vi "Example2.vi"() -> ()   [LabVIEW 2021]
doc: "Example of data acces and data flow in OOP in LabVIEW. Comments in Polish."
uses:
  Spaceship/Spaceship.lvclass
panel:
  out "Error Out 3":errorcluster
  out "Message Out 2":string
  out "Message Out":string
  in  "Spaceship.lvclass 2":refnum<class "Spaceship.lvclass">
  out "Error Out":errorcluster
  out "Error Out 2":errorcluster
  out "ID 2":string
  out "ID":string
  in  "Spaceship.lvclass":refnum<class "Spaceship.lvclass">
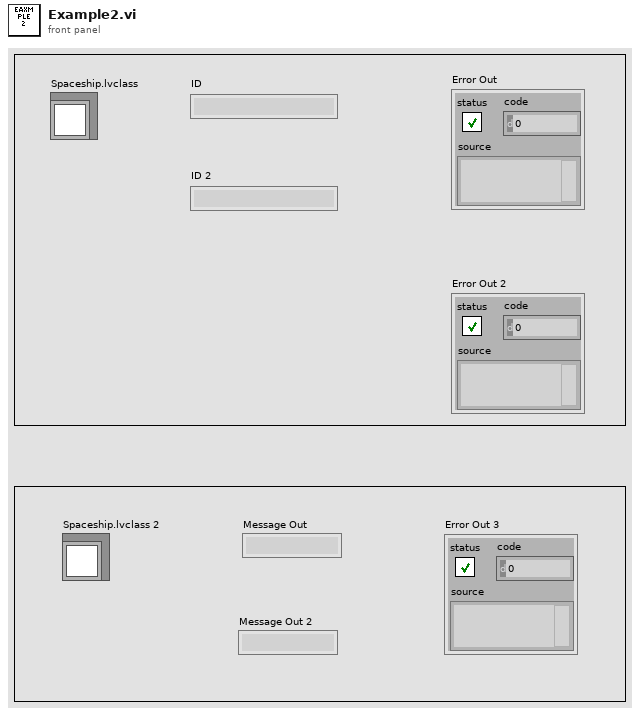
[diagram p1: front panel]
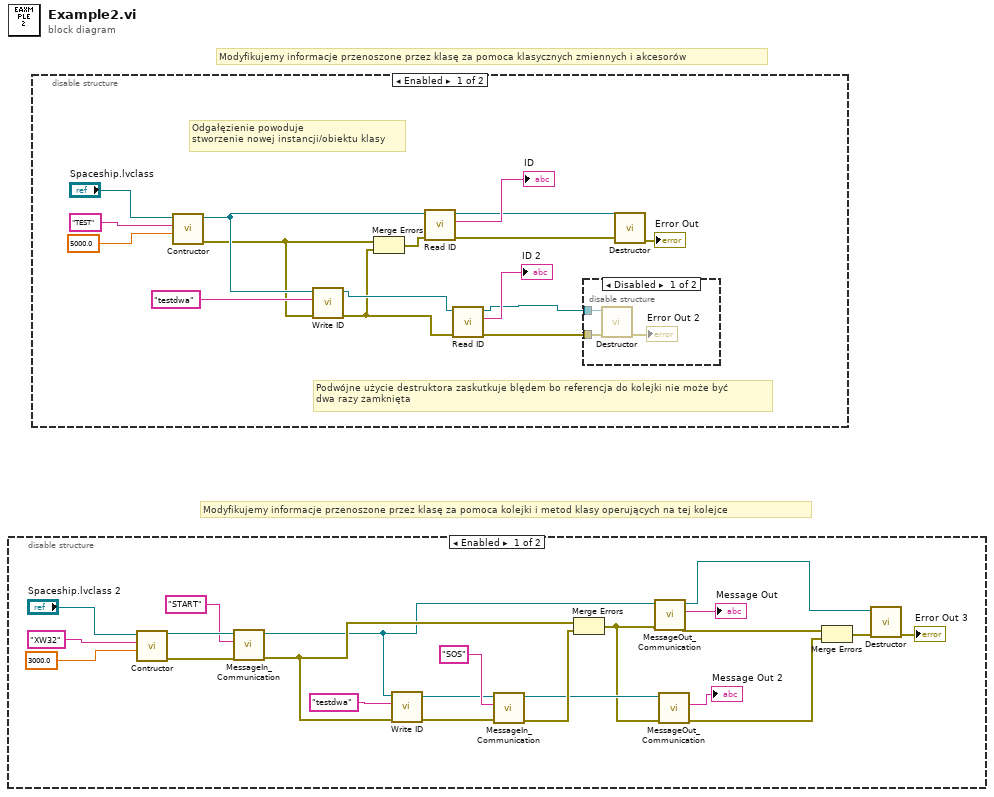
[diagram p0: block diagram]
diagram:
  # "Modyfikujemy informacje przenoszone przez klasę za pomoca kolejki i metod klasy operujących na tej kolejce"
  # "Modyfikujemy informacje przenoszone przez klasę za pomoca klasycznych zmiennych i akcesorów"
  n1 = disable-structure shown="Enabled" {
    frame Enabled {
      n2 = call-dynamic "Contructor.vi"("Speed [km/h]"=3000.0, "ID"="XW32", "Spaceship in"="Spaceship.lvclass 2") -> ("Error Out"=w18:errorcluster, "Spaceship out"=w19:refnum<class "Spaceship.lvclass">)  [unwired: 7 in]
      n3 = call-dynamic "MessageIn_Communication.vi"("Error In"=w18, "Message In"="START", "Spaceship in"=w19) -> ("Error Out"=w11:errorcluster, "Spaceship out"=w8:refnum<class "Spaceship.lvclass">)  [unwired: 7 in]
      n4 = call-dynamic "Write ID.vi"("error in (no error)"=w11, "ID"="testdwa", "Spaceship in"=w8) -> ("error out"=w14:errorcluster, "Spaceship out"=w13:refnum<class "Spaceship.lvclass">)  [unwired: 7 in]
      n5 = call-dynamic "MessageIn_Communication.vi"("Error In"=w14, "Message In"="SOS", "Spaceship in"=w13) -> ("Error Out"=w12:errorcluster, "Spaceship out"=w10:refnum<class "Spaceship.lvclass">)  [unwired: 7 in]
      n6 = Merge Errors(w11, w12) -> (w9:errorcluster)
      n7 = call-dynamic "MessageOut_Communication.vi"("Error In"=w9, "Spaceship in"=w8) -> ("Error Out"=w4:errorcluster, "Message Out"=→"Message Out":string, "Spaceship out"=w5:refnum<class "Spaceship.lvclass">)  [unwired: 7 in]
      n8 = call-dynamic "MessageOut_Communication.vi"("Error In"=w9, "Spaceship in"=w10) -> ("Error Out"=w2:errorcluster, "Message Out"=→"Message Out 2":string)  [unwired: 7 in, 1 out]
      n9 = Merge Errors(w4, w2) -> (w3:errorcluster)
      n10 = call-dynamic "Destructor.vi"("Error In"=w3, "Spaceship in"=w5) -> ("Error Out"=→"Error Out 3":errorcluster)  [unwired: 8 in, 1 out]
    }
    frame Disabled {
    }
  }
  n11 = disable-structure shown="Enabled" {
    frame Enabled {
      # "Podwójne użycie destruktora zaskutkuje blędem bo referencja do kolejki nie może być \ndwa razy zamknięta"
      # "Odgałęzienie powoduje\nstworzenie nowej instancji/obiektu klasy"
      n12 = call-dynamic "Contructor.vi"("Speed [km/h]"=5000.0, "ID"="TEST", "Spaceship in"="Spaceship.lvclass") -> ("Error Out"=w30:errorcluster, "Spaceship out"=w32:refnum<class "Spaceship.lvclass">)  [unwired: 7 in]
      n13 = call-dynamic "Write ID.vi"("error in (no error)"=w30, "ID"="testdwa", "Spaceship in"=w32) -> ("error out"=w27:errorcluster, "Spaceship out"=w28:refnum<class "Spaceship.lvclass">)  [unwired: 7 in]
      n14 = Merge Errors(w30, w27) -> (w29:errorcluster)
      n15 = call-dynamic "Read ID.vi"("error in (no error)"=w29, "Spaceship in"=w32) -> ("error out"=w34:errorcluster, "ID"=→"ID":string, "Spaceship out"=w33:refnum<class "Spaceship.lvclass">)  [unwired: 7 in]
      n16 = call-dynamic "Read ID.vi"("error in (no error)"=w27, "Spaceship in"=w28) -> ("error out"=w24:errorcluster, "ID"=→"ID 2":string, "Spaceship out"=w25:refnum<class "Spaceship.lvclass">)  [unwired: 7 in]
      n17 = disable-structure shown="Disabled" {
        disable-tunnel: w25 -> [w41 _]
        disable-tunnel: w24 -> [w40 _]
        frame Disabled {
          n18 = call-dynamic "Destructor.vi"("Error In"=w40, "Spaceship in"=w41) -> ("Error Out"=→"Error Out 2":errorcluster)  [unwired: 8 in, 1 out]
        }
        frame Enabled {
        }
      }
      n19 = call-dynamic "Destructor.vi"("Error In"=w34, "Spaceship in"=w33) -> ("Error Out"=→"Error Out":errorcluster)  [unwired: 8 in, 1 out]
    }
    frame Disabled {
    }
  }
